vi "TimeLeft.vi"(3 "Time Left":string) -> (0 "Completion":string)   [LabVIEW 2022 SP3]
panel:
  out "Seconds Left":i32
  out "Second":string
  out "Minute":string
  out "Hour":string
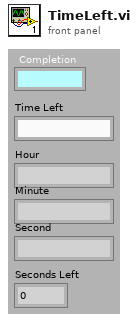
[diagram p1: front panel]
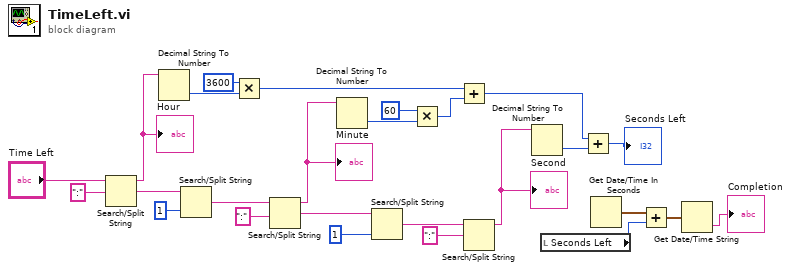
[diagram p0: block diagram]
diagram:
  n1 = Search/Split String(string="Time Left", search string/char (-)=":") -> (substring before match=w17:string, match + rest of string=w23:string)  [unwired: 1 in, 1 out]
  "Hour" <- w17
  n2 = Decimal String To Number(string=w17) -> (number=w13:i32)  [unwired: 2 in, 1 out]
  n3 = Search/Split String(string=w23, offset (0)=1) -> (match + rest of string=w25:string)  [unwired: 1 in, 2 out]
  n4 = Multiply(x=3600, y=w13) -> (x*y=w6:i32)
  n5 = Search/Split String(string=w25, search string/char (-)=":") -> (substring before match=w16:string, match + rest of string=w21:string)  [unwired: 1 in, 1 out]
  "Minute" <- w16
  n6 = Decimal String To Number(string=w16) -> (number=w11:i32)  [unwired: 2 in, 1 out]
  n7 = Search/Split String(string=w21, offset (0)=1) -> (match + rest of string=w19:string)  [unwired: 1 in, 2 out]
  n8 = Multiply(x=60, y=w11) -> (x*y=w10:i32)
  n9 = Add(x=w6, y=w10) -> (x+y=w7:i32)
  n10 = Search/Split String(string=w19, search string/char (-)=":") -> (substring before match=w15:string)  [unwired: 1 in, 2 out]
  "Second" <- w15
  n11 = Decimal String To Number(string=w15) -> (number=w1:i32)  [unwired: 2 in, 1 out]
  n12 = local read "Seconds Left"() -> (w4:i32)
  n13 = Add(x=w7, y=w1) -> (x+y=→"Seconds Left":i32)
  n14 = Get Date/Time In Seconds() -> (seconds since 1Jan1904=w5:timestamp)
  n15 = Add(x=w5, y=w4) -> (x+y=w3:timestamp)
  n16 = Get Date/Time String(seconds (now)=w3) -> (time string=→"Completion":string)  [unwired: 2 in, 1 out]
